vi "NMRvmeCard2.vi"() -> ()   [LabVIEW 2013]
uses:
  <vilib>/Utility/file.llb/Read From Spreadsheet File (DBL).vi
  <vilib>/Analysis/NI_AALBase.lvlib
panel:
  out "Telnet error out":errorcluster
  in  "Real/quad Q curve":bool=TRUE
  out "Temperature (C)":dbl(graph)=23.62
  out "+3V supply":dbl=3.245 format="%_4g"
  out "Temp (C)":dbl=23.62 format="%_4g"
  in  "RemovePed":bool=TRUE
  in  "IF / LOG Det":bool
  in  "Q curve file":string="realback213.txt"
  out "File name 2":string="C:\\users\\plm\\Desktop\\rssmt\\realback213.txt"
  in  "AutoBaseline":bool
  out "RF OK":bool=TRUE
  out "Peak area (V-MHz)":sgl=0.030135691 format="%.5f"
  in  "Gauss Fit":bool=TRUE
  out "NMR Graph + Fit":cluster{cluster{dbl, "Numeric":dbl}[]}[](graph)=[{[{212.6, "Numeric"=-0.007337857142857174}, {212.60999999999999, "Numeric"=0.0015661309523684781}, {212.62, "Numeric"=-0.006989880952367286}, {212.63, "Numeric"=-0.0018058928571413578}, {212.64, "Numeric"=-0.0008819047619148604}, {212.65, "Numeric"=-0.006517916666652648}, {212.66, "Numeric"=-0.004013928571425792}, {212.67, "Numeric"=0.004430059523801676}, {212.68, "Numeric"=-0.0036859523809383427}, {212.69, "Numeric"=-0.0025619642857105072}, {212.7, "Numeric"=-0.008197976190482105}, {212.71, "Numeric"=0.0062060119047757534}, {212.72, "Numeric"=-0.0010499999999954938}, {212.73, "Numeric"=0.005433988095233898}, {212.74, "Numeric"=0.007957976190462528}, {212.75, "Numeric"=-0.0004780357142806866}, {212.76, "Numeric"=0.002025952380949639}, {212.77, "Numeric"=0.00716994047617921}, {212.78, "Numeric"=0.004753928571433882}, {212.79, "Numeric"=0.005977916666665134}, {212.8, "Numeric"=0.0025419047618956726}, {212.81, "Numeric"=0.003145892857148176}, {212.82, "Numeric"=0.0028898809523804046}, {212.82999999999998, "Numeric"=-0.004626130952386719}, {212.84, "Numeric"=0.0025978571428622657}, {212.85, "Numeric"=0.0004618452380954173}, {212.85999999999999, "Numeric"=-0.0008341666666707862}, {212.87, "Numeric"=-0.005790178571423935}, {212.88, "Numeric"=0.0017938095238101666}, {212.89, "Numeric"=0.006917797619044916}, {212.9, "Numeric"=0.013381785714289643}, {212.91, "Numeric"=0.016685773809524684}, {212.92, "Numeric"=0.019929761904760382}, {212.93, "Numeric"=0.027013750000002956}, {212.94, "Numeric"=0.04453773809523895}, {212.95, "Numeric"=0.07450172619047558}, {212.96, "Numeric"=0.11950571428571606}, {212.97, "Numeric"=0.19734970238095298}, {212.98, "Numeric"=0.3199336904761906}, {212.99, "Numeric"=0.31055767857142735}, {213.0, "Numeric"=0.23802166666666674}, {213.01, "Numeric"=0.20112565476190528}, {213.02, "Numeric"=0.18826964285714298}, {213.03, "Numeric"=0.15635363095238028}, {213.04, "Numeric"=0.1528776190476197}, {213.05, "Numeric"=0.16054160714285845}, {213.06, "Numeric"=0.14854559523809352}, {213.07, "Numeric"=0.15518958333333396}, {213.08, "Numeric"=0.12887357142857359}, {213.09, "Numeric"=0.1011975595238066}, {213.1, "Numeric"=0.0636615476190479}, {213.11, "Numeric"=0.04466553571428848}, {213.12, "Numeric"=0.03580952380951938}, {213.13, "Numeric"=0.02519351190476165}, {213.14000000000001, "Numeric"=0.018317500000003165}, {213.15, "Numeric"=0.010081488095231909}, {213.16, "Numeric"=0.013485476190475125}, {213.17000000000002, "Numeric"=0.019629464285717615}, {213.18, "Numeric"=0.02171345238094422}, {213.19, "Numeric"=0.00043744047618837073}, {213.2, "Numeric"=0.004101428571433179}, {213.21, "Numeric"=-0.0027945833333437396}, {213.22, "Numeric"=-0.012250595238098632}, {213.23, "Numeric"=-0.005466607142852884}, {213.24, "Numeric"=0.004457380952392126}, {213.25, "Numeric"=-0.009078630952385888}, {213.26, "Numeric"=-0.011374642857139213}, {213.27, "Numeric"=-0.002630654761893246}, {213.28, "Numeric"=0.0011533333333266175}, {213.29, "Numeric"=-0.0075226785714257605}, {213.3, "Numeric"=-0.008658690476178892}, {213.31, "Numeric"=-0.000554702380961173}, {213.32, "Numeric"=0.004789285714287425}, {213.33, "Numeric"=-0.0019267261904647379}, {213.34, "Numeric"=-0.005302738095249119}, {213.35, "Numeric"=-0.01203874999999964}, {213.36, "Numeric"=0.0034652380952491305}, {213.37, "Numeric"=0.005309226190462615}, {213.38, "Numeric"=-0.0007067857142869088}, {213.39000000000001, "Numeric"=0.008017202380962745}, {213.4, "Numeric"=0.0012811904761741433}]}, {[{212.6, "Numeric"=4.477998384311765e-16}, {212.60999999999999, "Numeric"=2.2950395630551676e-15}, {212.62, "Numeric"=1.1297356240586014e-14}, {212.63, "Numeric"=5.3412619051196244e-14}, {212.64, "Numeric"=2.4254444205063017e-13}, {212.65, "Numeric"=1.0578380480827841e-12}, {212.66, "Numeric"=4.4312621479486125e-12}, {212.67, "Numeric"=1.7828553383592175e-11}, {212.68, "Numeric"=6.889459818419183e-11}, {212.69, "Numeric"=2.5570230350975336e-10}, {212.7, "Numeric"=9.11516453556325e-10}, {212.71, "Numeric"=3.1208635973986276e-09}, {212.72, "Numeric"=1.0262790552493904e-08}, {212.73, "Numeric"=3.2414292519770295e-08}, {212.74, "Numeric"=9.833045109131108e-08}, {212.75, "Numeric"=2.8649689468411557e-07}, {212.76, "Numeric"=8.01737522530931e-07}, {212.77, "Numeric"=2.154888996348111e-06}, {212.78, "Numeric"=5.562858336813754e-06}, {212.79, "Numeric"=1.3792770195388689e-05}, {212.8, "Numeric"=3.284622046080187e-05}, {212.81, "Numeric"=7.512763364390388e-05}, {212.82, "Numeric"=0.00016504197766844557}, {212.82999999999998, "Numeric"=0.00034823268507752647}, {212.84, "Numeric"=0.0007057080104084037}, {212.85, "Numeric"=0.0013736021621510133}, {212.85999999999999, "Numeric"=0.0025678951530750086}, {212.87, "Numeric"=0.004610775878464986}, {212.88, "Numeric"=0.007951538031376609}, {212.89, "Numeric"=0.013170694359882934}, {212.9, "Numeric"=0.020953018953416967}, {212.91, "Numeric"=0.03201584311771621}, {212.92, "Numeric"=0.046985481701043365}, {212.93, "Numeric"=0.06622818103081612}, {212.94, "Numeric"=0.08966075135486304}, {212.95, "Numeric"=0.11658490515295523}, {212.96, "Numeric"=0.14560043639077294}, {212.97, "Numeric"=0.17464792601848012}, {212.98, "Numeric"=0.2012076977407145}, {212.99, "Numeric"=0.2226415178154416}, {213.0, "Numeric"=0.23661818536763396}, {213.01, "Numeric"=0.24152966994721356}, {213.02, "Numeric"=0.2367953988974436}, {213.03, "Numeric"=0.2229751343039549}, {213.04, "Numeric"=0.2016601156875433}, {213.05, "Numeric"=0.17517171944390159}, {213.06, "Numeric"=0.14614648582469741}, {213.07, "Numeric"=0.11710977972798974}, {213.08, "Numeric"=0.09013186434319223}, {213.09, "Numeric"=0.06662603179824521}, {213.1, "Numeric"=0.047303137158804374}, {213.11, "Numeric"=0.03225643326293323}, {213.12, "Numeric"=0.021126285598009813}, {213.13, "Numeric"=0.01328955235357364}, {213.14000000000001, "Numeric"=0.008029305111634542}, {213.15, "Numeric"=0.004659356849703404}, {213.16, "Numeric"=0.0025968949900007465}, {213.17000000000002, "Numeric"=0.001390154938300592}, {213.18, "Numeric"=0.0007147471432035038}, {213.19, "Numeric"=0.0003529572058190503}, {213.2, "Numeric"=0.00016740640890758706}, {213.21, "Numeric"=7.626100266986159e-05}, {213.22, "Numeric"=3.336670677946763e-05}, {213.23, "Numeric"=1.402182626664142e-05}, {213.24, "Numeric"=5.659475991032893e-06}, {213.25, "Numeric"=2.193957775883827e-06}, {213.26, "Numeric"=8.168846048211217e-07}, {213.27, "Numeric"=2.9212825246695113e-07}, {213.28, "Numeric"=1.0033831723559814e-07}, {213.29, "Numeric"=3.310095080967592e-08}, {213.3, "Numeric"=1.0488044650570882e-08}, {213.31, "Numeric"=3.191750899512875e-09}, {213.32, "Numeric"=9.329188202520945e-10}, {213.33, "Numeric"=2.619021854862434e-10}, {213.34, "Numeric"=7.061789920050181e-11}, {213.35, "Numeric"=1.8288196018066986e-11}, {213.36, "Numeric"=4.548910010060871e-12}, {213.37, "Numeric"=1.0867364300189267e-12}, {213.38, "Numeric"=2.4935696854046353e-13}, {213.39000000000001, "Numeric"=5.495398568628478e-14}, {213.4, "Numeric"=1.1632077475457075e-14}]}]
  in  "Amp of Q curve":dbl=1.8000000000000005 min=0.0 max=7.0 step=0.01 format="%_3f"
  in  "Subtract Q curve":bool=TRUE
  in  "Adjust Tune":bool
  out "Pedestal Offset":dbl(graph)=0.11233333333333334
  out "Pedestal Difference":dbl(graph)=0.027776666666669073
  out "# Good Spectra":i32=8751
  in  "Quality cuts":bool=TRUE
  out "Pedestal OK":bool=TRUE
  out "Sweep #":i32=9576
  out "1st Sweep":bool
  out "ADC volts OK":bool=TRUE
  out "Peak Height Distribution":cluster{"Y":dbl[], "Y":dbl[]}[](graph)=[{"Y"=[0.20096167468517595, 0.20217254526145662, 0.20338341583773728, 0.20459428641401792, 0.20580515699029858, 0.20701602756657925, 0.2082268981428599, 0.20943776871914058, 0.21064863929542121, 0.21185950987170188, 0.21307038044798254, 0.2142812510242632, 0.21549212160054387, 0.21670299217682454, 0.21791386275310518, 0.21912473332938584, 0.2203356039056665, 0.22154647448194717, 0.22275734505822783, 0.22396821563450847, 0.22517908621078914, 0.2263899567870698, 0.22760082736335047, 0.22881169793963113, 0.2300225685159118, 0.23123343909219243, 0.2324443096684731, 0.23365518024475376, 0.23486605082103443, 0.2360769213973151, 0.23728779197359576, 0.2384986625498764, 0.23970953312615706, 0.24092040370243772, 0.2421312742787184, 0.24334214485499905, 0.2445530154312797, 0.24576388600756036, 0.24697475658384102, 0.24818562716012169, 0.24939649773640235, 0.250607368312683, 0.25181823888896365, 0.2530291094652443, 0.254239980041525, 0.25545085061780565, 0.2566617211940863, 0.257872591770367, 0.25908346234664764, 0.2602943329229283, 0.2615052034992089, 0.2627160740754896, 0.26392694465177025, 0.2651378152280509, 0.2663486858043316, 0.26755955638061224, 0.2687704269568929, 0.26998129753317357, 0.27119216810945423, 0.2724030386857349, 0.27361390926201556, 0.2748247798382962, 0.27603565041457684, 0.2772465209908575, 0.27845739156713817, 0.27966826214341883, 0.2808791327196995, 0.28209000329598016, 0.2833008738722608, 0.2845117444485415, 0.28572261502482216, 0.2869334856011028, 0.28814435617738343, 0.2893552267536641, 0.29056609732994476, 0.2917769679062254, 0.2929878384825061, 0.29419870905878676, 0.2954095796350674, 0.2966204502113481, 0.29783132078762875, 0.2990421913639094, 0.3002530619401901, 0.3014639325164707, 0.30267480309275135, 0.303885673669032, 0.3050965442453127, 0.30630741482159335, 0.307518285397874, 0.3087291559741547, 0.30994002655043534, 0.311150897126716, 0.3123617677029967, 0.31357263827927734, 0.31478350885555795, 0.3159943794318386, 0.3172052500081193, 0.31841612058439994, 0.3196269911606806, 0.32083786173696127], "Y"=[1.0, 1.0, 1.0, 1.0, 1.0, 3.0, 1.0, 3.0, 12.0, 14.0, 11.0, 33.0, 21.0, 34.0, 39.0, 52.0, 67.0, 81.0, 110.0, 118.0, 144.0, 149.0, 197.0, 195.0, 243.0, 257.0, 288.0, 310.0, 311.0, 354.0, 388.0, 378.0, 397.0, 413.0, 404.0, 387.0, 378.0, 337.0, 341.0, 295.0, 284.0, 270.0, 218.0, 192.0, 181.0, 167.0, 129.0, 100.0, 88.0, 103.0, 56.0, 45.0, 26.0, 28.0, 36.0, 18.0, 16.0, 2.0, 8.0, 4.0, 2.0, 2.0, 0.0, 2.0, 1.0, 0.0, 0.0, 0.0, 0.0, 0.0, 0.0, 0.0, 0.0, 0.0, 0.0, 0.0, 0.0, 0.0, 0.0, 0.0, 0.0, 0.0, 0.0, 0.0, 0.0, 0.0, 0.0, 0.0, 0.0, 0.0, 0.0, 0.0, 0.0, 0.0, 0.0, 0.0, 0.0, 0.0, 0.0, 3.0]}]
  in  "# of Sweeps":i32=10000
  out "S/N":dbl=22.210089077083225 format="%_3g"
  out "Peak mean (V)":dbl=0.2407315251032532 format="%_4g"
  out "Peak Height":dbl(graph)=0.24153008942931342
  in  "Raw Data":bool=TRUE
  in  "Tank RF":bool=TRUE
  in  "IF Atten (dB)":i8=3 min=0 max=31 step=1
  in  "IFoffset (V)":dbl=5.361519 min=-0.0 max=9.0 step=0.001 format="%.4f"
  in  "Tune  (V)":dbl=0.3399666666666663 min=0.0 max=5.0 step=0.001 format="%.4f"
  in  "Hi / Lo IF Gain":bool
  out "Voltage Array":sgl[](array[numeric])=[0.3804, 0.3754, 0.3533, 0.3453, 0.3334, 0.3153, 0.3057, 0.3024, 0.2829, 0.273, 0.2567, 0.2608, 0.2436, 0.2405, 0.2338, 0.2165, 0.2105, 0.2075, 0.1973, 0.1911, 0.1806, 0.1745, 0.1679, 0.1544, 0.156, 0.1486, 0.1424, 0.1329, 0.1363, 0.1376, 0.1406, 0.1408, 0.1413, 0.146, 0.1615, 0.1898, 0.2335, 0.3104, 0.4324, 0.4228, 0.3504, 0.314, 0.302, 0.2713, 0.2694, 0.279, 0.2693, 0.2786, 0.2553, 0.231, 0.1972, 0.1823, 0.1779, 0.1721, 0.1704, 0.1677, 0.177, 0.1894, 0.1981, 0.1838, 0.1948, 0.1956, 0.1942, 0.2094, 0.2281, 0.2237, 0.2309, 0.2495, 0.2635, 0.2654, 0.2752, 0.2946, 0.3116, 0.3169, 0.3259, 0.3319, 0.3605, 0.3758, 0.3836, 0.4065, 0.4143] format="%.4f"
  in  "Invert Polarity":bool=TRUE
  out "Pedestal Diff (V)":sgl=0.027776666 format="%.3f"
  out "Peak amp (V)":sgl=0.24153009 format="%.3f"
  in  "Save Data to File":bool
  in  "RF Level (dBm)":dbl min=-10.0 max=10.0 step=0.1 format="%.2f"
  out "SMT error out":errorcluster
  out "Sample RMS (V)":dbl=0.00852469135802469 format="%.4f"
  in  "# Sample/step":i32=80 min=1 max=1000 step=100
  in  "Step Width (MHz)":dbl=0.01 min=0.0 max=1000.0 step=0.0005 format="%.4f"
  in  "Freq Span (MHz)":dbl=0.8 min=0.0 max=3000.0 step=0.1 format="%.3f"
  in  "Center Freq (MHz)":dbl=213.0 min=0.005 max=6000.0 step=0.1 format="%.3f"
  in  "Sweep Mode":u16(ring)=3 items=["Off", "Single", "Auto", "Step"]
  in  "GPIB Addr (28)":refnum<visa-resource-name>="GPIB0::28::INSTR"
  # "E1039 Prototype NMR Control Panel"
  # "Settings"
  # "D\nA\nC"
  # "R\nF\n\nG\nE\nN \n\n+\n\nI\nF"
  # "A\nD\nC"
  # "D\nA\nT\nA\n\n+\n\nA \nN\nA\nL\nY\nS\nI\nS"
  # "I\n/\nO"
  # "Results"
  # "A\nv\ne\nr\na\ng\ne"
  # "S\nw\ne\ne\np"
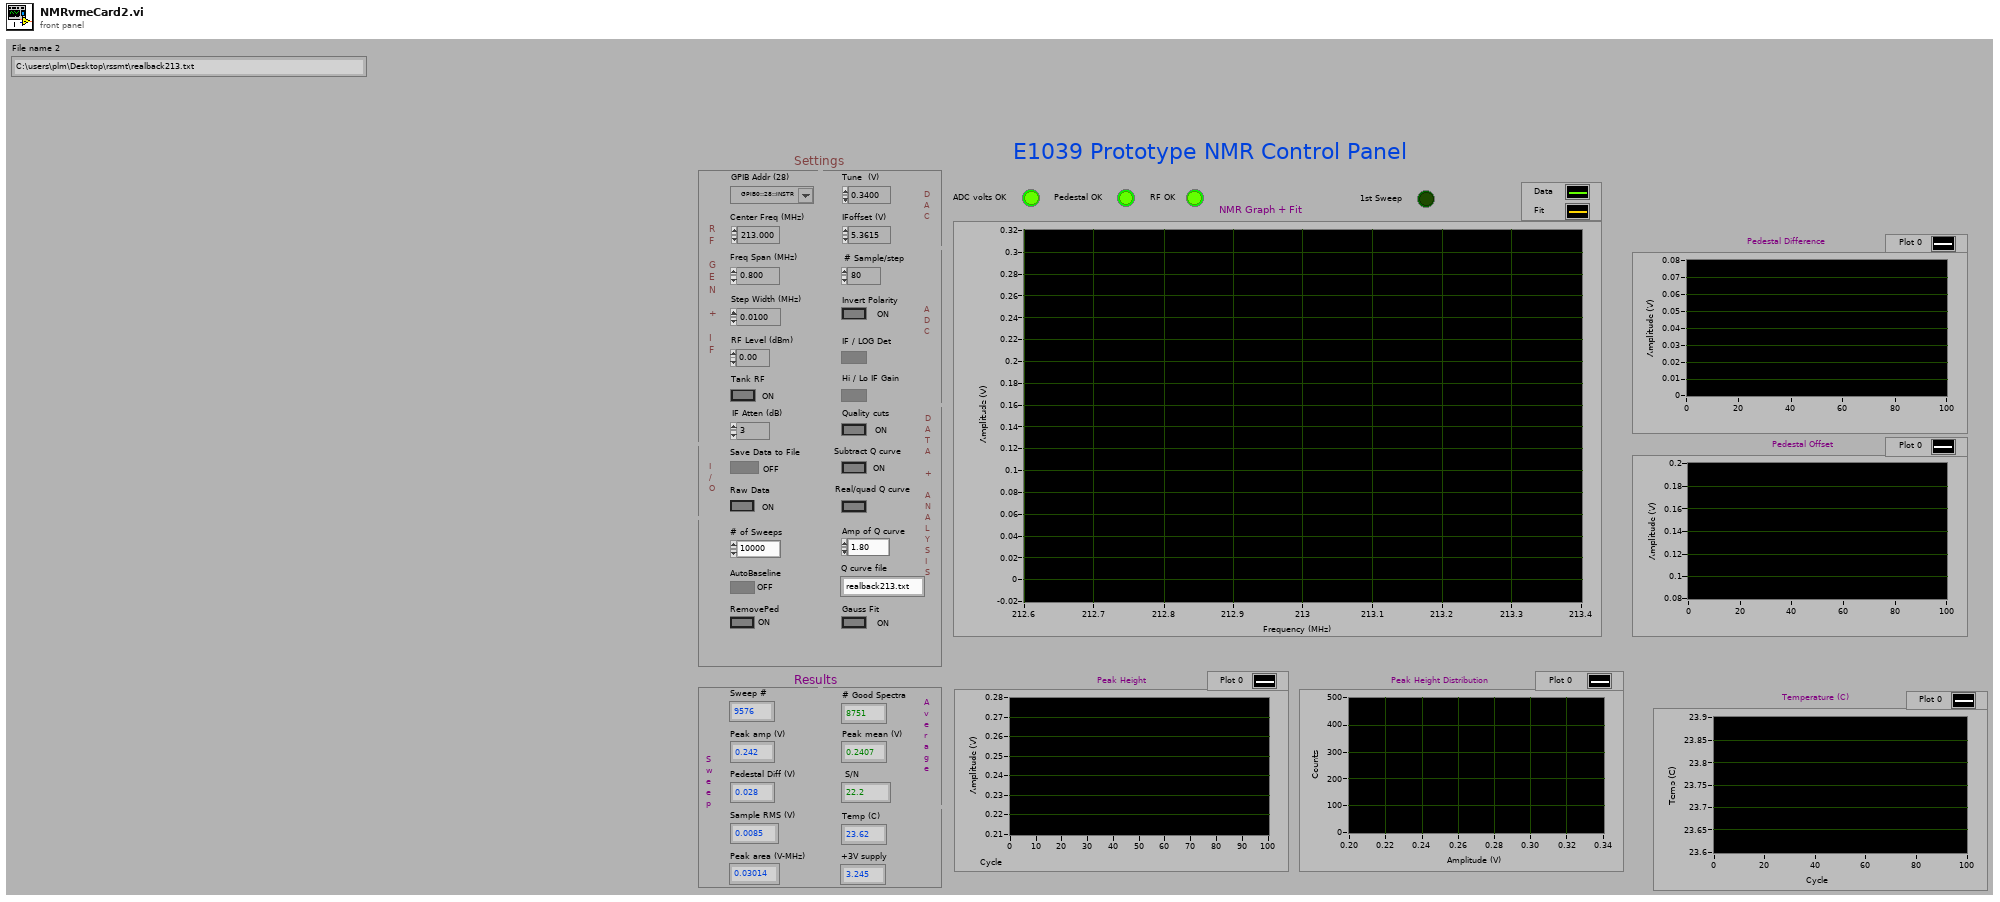
[diagram p1: front panel]
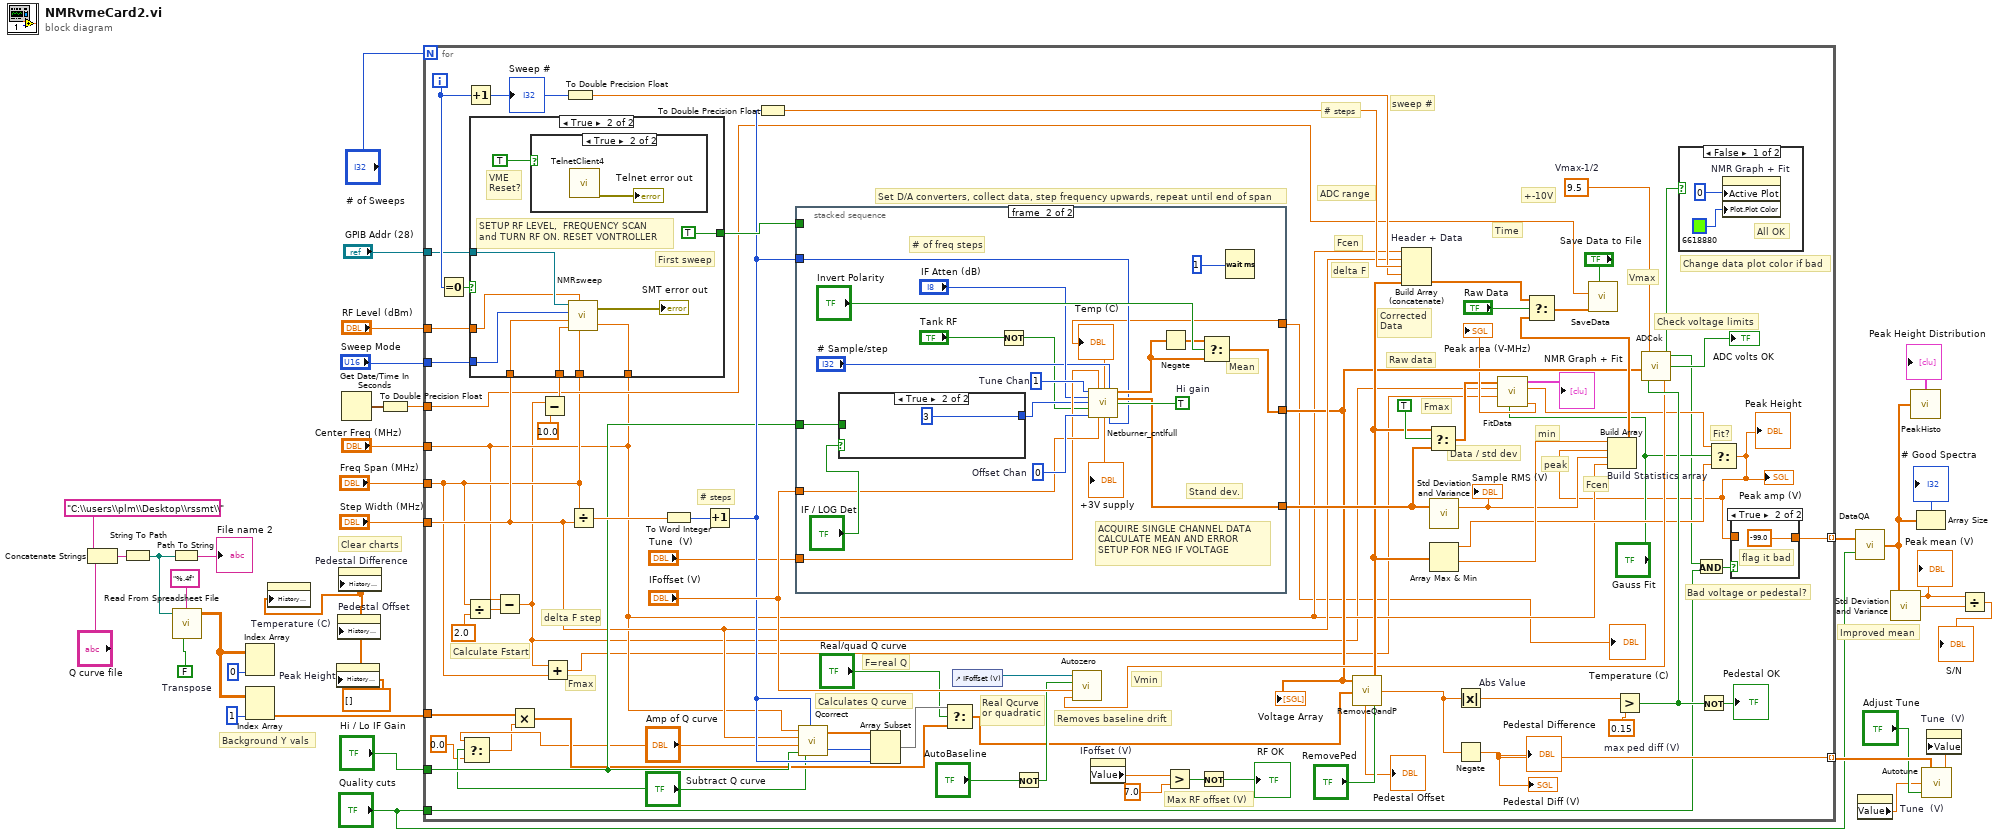
[diagram p0: block diagram]
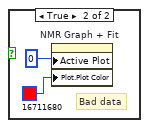
[diagram p2: hidden frame]
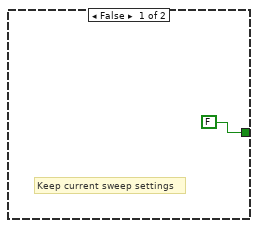
[diagram p4: hidden frame]
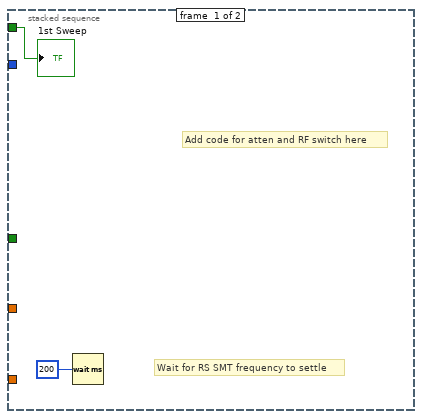
[diagram p6: hidden frame]
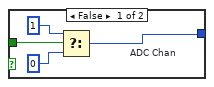
[diagram p7: hidden frame]
diagram:
  w12 = FALSE  # Transpose
  w4 = dbl[] []
  # "Background Y vals"
  # "Clear charts"
  # "Improved mean"
  n1 = Concatenate Strings "Concatenate Strings"("C:\\users\\plm\\Desktop\\rssmt\\", "Q curve file") -> (w15:string)
  n2 = String To Path(string=w15) -> (path=w11:path)
  n3 = Path To String(path=w11) -> (string=→"File name 2":string)
  n4 = call-poly <vilib>:"Read From Spreadsheet File.vi"("transpose (no:F)"=w12, "format (%.3f)"="%.4f", "file path (dialog if empty)"=w11) -> ("all rows"=w10:dbl[][])  [unwired: 4 in, 4 out]
  n5 = Index Array "Index Array"(array=w10, index (col)=0) -> ()  [unwired: 1 in, 1 out]
  n6 = Index Array(array=w10, index (col)=1) -> (element=w5:dbl[])  [unwired: 1 in]
  n7 = property on="Temperature (C)" class="WFChart (strict)"("History Data"=w4) -> ()  [unwired: 2 in, 2 out]
  n8 = property on="Peak Height" class="WFChart (strict)"("History Data"=w4) -> ()  [unwired: 2 in, 2 out]
  n9 = property on="Pedestal Offset" class="WFChart (strict)"("History Data"=w4) -> ()  [unwired: 2 in, 2 out]
  n10 = property on="Pedestal Difference" class="WFChart (strict)"("History Data"=w4) -> ()  [unwired: 2 in, 2 out]
  n11 = Get Date/Time In Seconds() -> (seconds since 1Jan1904=w17:timestamp)
  n12 = To Double Precision Float(number=w17) -> (double precision float=w16:dbl)
  n13 = for {
    N: "# of Sweeps" -> [_]
    tunnel: [w95] -> w32 mode=indexing
    tunnel: "Quality cuts" -> [w72]
    tunnel: [w78] -> w29 mode=indexing
    tunnel: "Center Freq (MHz)" -> [w59]
    tunnel: "Freq Span (MHz)" -> [w65]
    tunnel: "Step Width (MHz)" -> [w71]
    tunnel: "Sweep Mode" -> [w82]
    tunnel: "Hi / Lo IF Gain" -> [w81]
    tunnel: "GPIB Addr (28)" -> [w80]
    tunnel: "RF Level (dBm)" -> [w79]
    tunnel: w16 -> [w66]
    tunnel: w5 -> [w44]
    i -> [w93]
    w76 = 9.5  # Vmax-1/2
    w96 = 0.15  # max ped diff (V)
    # "F=real Q"
    # "Real Qcurve\nor quadratic"
    # "+-10V"
    # "Vmax"
    # "Change data plot color if bad"
    # "Max RF offset (V)"
    # "Fmax"
    # "Fit?"
    # "Fmax"
    # "Time"
    # "Vmin"
    # "min"
    # "peak"
    # "Raw data"
    # "Corrected\nData"
    # "Fcen"
    # "delta F"
    # "# steps"
    # "ADC range"
    # "sweep #"
    # "Fcen"
    # "Set D/A converters, collect data, step frequency upwards, repeat until end of span"
    # "Calculates Q curve"
    # "Removes baseline drift"
    # "Bad voltage or pedestal?"
    # "Check voltage limits"
    # "Data / std dev"
    # "# steps"
    # "Calculate Fstart"
    # "delta F step"
    n14 = Equal To 0?(x=w93) -> (x = 0?=w98:bool)
    n15 = Select(t="Amp of Q curve", s="Subtract Q curve", f=0.0) -> (s? t:f=w39:dbl)
    n16 = Divide(x=w65, y=sgl 2.0) -> (x/y=w109:dbl)
    n17 = Increment(x=w93) -> (x+1=w83:i32)
    "Sweep #" <- w83
    n18 = Subtract(x=w59, y=w109) -> (x-y=w54:dbl)
    n19 = Multiply(x=w44, y=w39) -> (x*y=w43:dbl[])
    n20 = Subtract(x=w54, y=10.0) -> (x-y=w107:dbl)
    n21 = case shown="True" w98 {
      tunnel: w107 -> [_ w128]
      tunnel: w71 -> [_ w126]
      tunnel: w59 -> [_ w125]
      tunnel: w65 -> [_ w127]
      tunnel: [FALSE TRUE] -> w97
      tunnel: w82 -> [_ w122]
      tunnel: w80 -> [_ w121]
      tunnel: w79 -> [_ w120]
      frame False {
        # "Keep current sweep settings"
      }
      frame True {
        # "VME\nReset?"
        # "First sweep"
        # "SETUP RF LEVEL,  FREQUENCY SCAN\nand TURN RF ON. RESET VONTROLLER"
        n22 = case shown="True" TRUE {
          frame False {
          }
          frame True {
            n23 = call "TelnetClient4.vi"() -> ("Telnet error"=→"Telnet error out":errorcluster)  [unwired: 4 in, 3 out]
          }
        }
        n24 = call "NMRsweep.vi"("Center Freq (MHz)"=w125, "Freq Span (MHz)"=w127, "RF Level (dBm)"=w120, "Foffset (MHz)"=w128, "Step Width (MHz)"=w126, "Sweep Mode"=w122, "GPIB Addr (28)"=w121) -> ("error out"=→"SMT error out":errorcluster)
      }
    }
    n25 = Add(x=w54, y=w65) -> (x+y=w53:dbl)
    n26 = To Double Precision Float(number=w83) -> (double precision float=w84:dbl)
    n27 = Divide(x=w65, y=w71) -> (x/y=w111:dbl)
    n28 = To Word Integer(number=w111) -> (16bit integer=w108:i16)
    n29 = Increment(x=w108) -> (x+1=w87:i16)
    n30 = To Double Precision Float(number=w87) -> (double precision float=w86:dbl)
    n31 = stacked-sequence {
      tunnel: [_ w139] -> w101
      tunnel: [_ w150] -> w69
      tunnel: w87 -> [_ w136]
      tunnel: "IFoffset (V)" -> [_ w145]
      tunnel: w81 -> [_ w148]
      tunnel: w97 -> [w130 _]
      tunnel: "Tune  (V)" -> [_ w143]
      tunnel: [_ w134] -> w35
      frame #0 {
        # "Add code for atten and RF switch here"
        # "Wait for RS SMT frequency to settle"
        n32 = Wait (ms)(milliseconds to wait=200) -> ()  [unwired: 1 out]
        "1st Sweep" <- w130
      }
      frame #1 {
        w141 = TRUE  # Hi gain
        w146 = 0  # Offset Chan
        w144 = 1  # Tune Chan
        # "Stand dev."
        # "Mean"
        # "ACQUIRE SINGLE CHANNEL DATA\nCALCULATE MEAN AND ERROR\nSETUP FOR NEG IF VOLTAGE"
        # "# of freq steps"
        n33 = case shown="True" "IF / LOG Det" {
          tunnel: w148 -> [w156 _]
          tunnel: [w153 3] -> w138
          frame False {
            n34 = Select "ADC Chan"(t=1, s=w156, f=0) -> (s? t:f=w153:i32)
          }
          frame True {
          }
        }
        n35 = Not(x="Tank RF") -> (.not. x?=w133:bool)
        n36 = call "Netburner_cntlfull.vi"("Tune DAC"=w144, "Tune Volt"=w143, "# Data"="# Sample/step", "IF Atten (dB)"="IF Atten (dB)", "NMR ADC"=w138, "Hi Gain"=w141, "Tank RF"=w133, "Offset DAC"=w146, "Offset Volt"=w145, "# f steps"=w136) -> ("Temp (C)"=w134:dbl, "ADC value"=w140:dbl[], "ADC error"=w139:dbl[], "Volts"=→"+3V supply":dbl)  [unwired: 2 out]
        "Temp (C)" <- w134
        n37 = Negate(x=w140) -> (-x=w149:dbl[])
        n38 = Select(t=w149, s="Invert Polarity", f=w140) -> (s? t:f=w150:dbl[])
        n39 = Wait (ms)(milliseconds to wait=1) -> ()  [unwired: 1 out]
      }
    }
    "Voltage Array" <- w69
    "Temperature (C)" <- w35
    n40 = call "Qcorrect.vi"("Subtract Q curve"="Subtract Q curve", "Nstep"=w87, "IF or Log"=w81, "Amp of Q curve"="Amp of Q curve", "Step Width (MHz)"=w71, "Center Freq (MHz)"=w59) -> ("Start"=w102:i32, "Array"=w103:dbl[])
    n41 = Array Subset "Array Subset"(array=w103, index=w102, length=w87) -> (w47:dbl[])
    n42 = Select(t=w47, s="Real/quad Q curve", f=w43) -> (s? t:f=w46:dbl[])
    n43 = control-ref of="IFoffset (V)"() -> (w75:refnum<vi>)
    n44 = Not(x="AutoBaseline") -> (.not. x?=w48:bool)
    n45 = property on="IFoffset (V)" class="DigNum (strict)"() -> ("Value"=w63:dbl)  [unwired: 2 in, 2 out]
    n46 = Greater?(x=w63, y=7.0) -> (0:w61:bool)
    n47 = Not(x=w61) -> (.not. x?=→"RF OK":bool)
    n48 = call "RemoveQandP.vi"("Subtract Ped?"="RemovePed", "Qcurve"=w46, "Raw data"=w69) -> ("Ped L-R"=w89:dbl, "Corrected data"=w85:dbl[], "Ped Offfset"=→"Pedestal Offset":dbl)
    n49 = Build Array (concatenate) "Header + Data"(w59, w71, w86, w84, w85) -> (w88:dbl[])
    n50 = Select(t=w85, s=TRUE, f=w101) -> (s? t:f=w55:dbl[])
    n51 = call <vilib>:"Std Deviation and Variance.vi"("X"=w101) -> ("mean"=w70:dbl)  [unwired: 1 in, 2 out]
    "Sample RMS (V)" <- w70
    n52 = Array Max & Min(array=w85) -> (max value=w64:dbl, min value=w100:dbl)  [unwired: 2 out]
    n53 = Absolute Value "Abs Value"(x=w89) -> (abs(x)=w91:dbl)
    n54 = Negate(x=w89) -> (-x=w78:dbl)
    "Pedestal Diff (V)" <- w78
    "Pedestal Difference" <- w78
    n55 = call "FitData.vi"("Fit?"="Gauss Fit", "Fmax"=w53, "Fmin"=w54, "Yarray"=w55) -> ("Peak Area (V-MHz)"=→"Peak area (V-MHz)":dbl, "Amplitude (V)"=w57:dbl, "NMR Graph + Fit"=→"NMR Graph + Fit":cluster{cluster{dbl, "Numeric":dbl}[]}[])  [unwired: 2 out]
    n56 = Greater?(x=w91, y=w96) -> (0:w77:bool)
    n57 = call "ADCok.vi"("PedOK"=w77, "Array"=w69, "Vmax-1/2"=w76) -> ("Vmin"=w74:dbl, "ADC voltages OK"=→"ADC volts OK":bool, "Allok"=w51:bool)
    n58 = call "Autozero.vi"("Vmin (V)"=w74, "IFoffset (V)"="IFoffset (V)", "IF or Log"=w48, "reference"=w75) -> ()
    n59 = case shown="False" w51 {
      frame False {
        # "All OK"
        n60 = property on="NMR Graph + Fit" class="XYGraph (strict)"("Active Plot"=0, "Plot.Plot Color"=u32 6618880) -> ()  [unwired: 2 in, 2 out]
      }
      frame True {
        # "Bad data"
        n61 = property on="NMR Graph + Fit" class="XYGraph (strict)"("Active Plot"=0, "Plot.Plot Color"=u32 16711680) -> ()  [unwired: 2 in, 2 out]
      }
    }
    n62 = And(x=w51, y=w72) -> (x .and. y?=w92:bool)
    n63 = Not(x=w77) -> (.not. x?=→"Pedestal OK":bool)
    n64 = Select(t=w57, s="Gauss Fit", f=w64) -> (s? t:f=w50:dbl)
    "Peak amp (V)" <- w50
    "Peak Height" <- w50
    n65 = Build Array "Build Statistics array"(w100, w50, w70, w59) -> (w106:dbl[])
    n66 = Select(t=w88, s="Raw Data", f=w106) -> (s? t:f=w67:dbl[])
    n67 = call "SaveData.vi"("Array"=w67, "Save Data to File"="Save Data to File", "Ext time (sec)"=w66) -> ()  [unwired: 1 out]
    n68 = case shown="True" w92 {
      tunnel: [w116 -99.0] -> w95
      tunnel: w50 -> [w116 _]
      frame False {
        # "Data OK"
      }
      frame True {
        # "flag it bad"
      }
    }
  }
  n69 = call "DataQA.vi"("Quality cuts"="Quality cuts", "Data In"=w32) -> ("Data Out"=w31:dbl[])
  n70 = property on="Tune  (V)" class="DigNum (strict)"() -> ("Value"=w20:dbl)  [unwired: 2 in, 2 out]
  n71 = call <vilib>:"Std Deviation and Variance.vi"("X"=w31) -> ("mean"=w3:dbl, "standard deviation"=w2:dbl)  [unwired: 1 in, 1 out]
  "Peak mean (V)" <- w3
  n72 = call "PeakHisto.vi"("Data Out"=w31) -> ("XY Graph"=→"Peak Height Distribution":cluster{"Y":dbl[], "Y":dbl[]}[])
  n73 = Array Size(array=w31) -> (size(s)=→"# Good Spectra":i32)
  n74 = call "Autotune.vi"("Adjust Tune"="Adjust Tune", "Tune Vin"=w20, "Pedestal Diff"=w29) -> ("Tune Vout"=w19:dbl)
  n75 = property on="Tune  (V)" class="DigNum (strict)"("Value"=w19) -> ()  [unwired: 2 in, 2 out]
  n76 = Divide(x=w3, y=w2) -> (x/y=→"S/N":dbl)
